vi "GT Load Ext Config.vi"(8 "error in (no error)":errorcluster caption="错误输入（无错误）", 10 "pFileName":string, 11 "cardNum":i16) -> (0 "error out":errorcluster caption="错误输出", 2 "pFileName out":string, 3 "function return":i16)   [LabVIEW 2020, in "gts.lvlib"]
doc: "GT_API GT_LoadExtConfig(short cardNum,char *pFileName);"
uses:
  gts.lvlib
  dll/32bit/multi_card/gts.dll
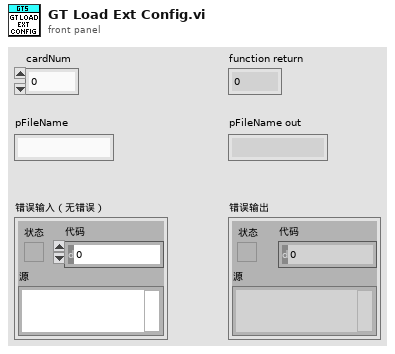
[diagram p1: front panel]
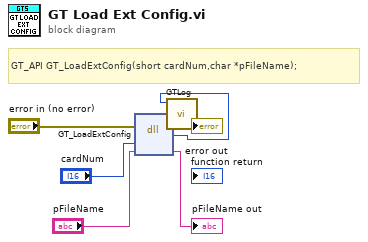
[diagram p0: block diagram]
diagram:
  # "GT_API GT_LoadExtConfig(short cardNum,char *pFileName);"
  n1 = dll-call lib="C:/1228/dll/32bit/multi_card/gts.dll" fn="GT_LoadExtConfig"(error in="error in (no error)", "cardNum"="cardNum", "pFileName"="pFileName") -> (error out=w3:errorcluster, w1:i16, "pFileName"=→"pFileName out":string)  [unwired: 3 in, 1 out]
  n2 = call "GTLog.vi"("error in (no error)"=w3, "Numeric"=w1) -> ("error out"=→"error out":errorcluster)  [unwired: 9 in]
